vi "Get Array Values as JSON.vi"(8 "error in (no error)":errorcluster, 11 "JSON Array in":refnum<class "JSON Array.lvclass">) -> (0 "error out":errorcluster, 1 "single type?":bool, 2 "types":T1[](array[typedef]), 3 "values":refnum<class "JSON Null.lvclass">[](array[class]))   [LabVIEW 2016, in "LVJSON.lvlib" / "JSON Array.lvclass"]
doc: "Returns the element type of each element in a JSON Array. If all elements are of the same type, single type is true."
uses:
  JSON Array.lvclass
  JSON Types.ctl
  JSON Datatype/JSON Null.lvclass
  JSON Array.lvclass/JSON Array.ctl
  LVJSON.lvlib
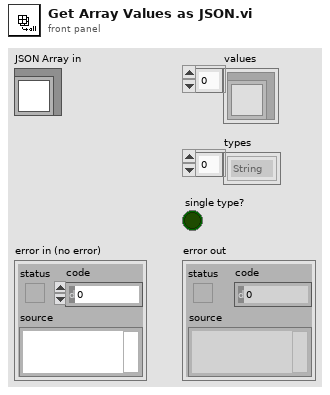
[diagram p1: front panel]
types:
  T1 = typedef "LVJSON.lvlib/JSON Types.ctl" = enum16{"String", "Numeric", "Boolean", "NULL", "Object", "Array"}
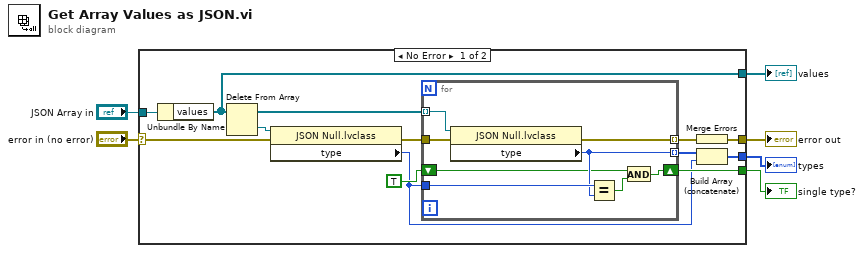
[diagram p0: block diagram]
diagram:
  n1 = case shown="No Error" "error in (no error)" {
    selector: "error in (no error)" -> [w11 w28]
    tunnel: [w8 w28] -> w5
    tunnel: "JSON Array in" -> [w19 _]
    tunnel: [w13 _] -> w3
    tunnel: [w15 _] -> w2
    tunnel: [w7 _] -> w1
    frame No Error {
      n2 = Unbundle By Name(w19) -> ("values"=w7:refnum<class "JSON Null.lvclass">[])
      n3 = Delete From Array(array=w7) -> (deleted portion=w18:refnum<class "JSON Null.lvclass">, array with subset deleted=w17:refnum<class "JSON Null.lvclass">[])  [unwired: 2 in]
      n4 = property class="JSON Null.lvclass"(reference=w18, error in=w11) -> (error out=w10:errorcluster, "type"=w12:T1)  [unwired: 1 out]
      n5 = for {
        tunnel: w17 -> [w27] mode=indexing
        tunnel: [w25] -> w14 mode=indexing
        tunnel: w12 -> [w26]
        shift-right: [w22] -> w15
        shift-left: TRUE -> [w23]
        tunnel: w10 -> [w21]
        tunnel: [w20] -> w9 mode=indexing
        n6 = property class="JSON Null.lvclass"(reference=w27, error in=w21) -> (error out=w20:errorcluster, "type"=w25:T1)  [unwired: 1 out]
        n7 = Equal?(x=w26, y=w25) -> (x = y?=w24:bool)
        n8 = And(x=w23, y=w24) -> (x .and. y?=w22:bool)
      }
      n9 = Merge Errors(w9) -> (w8:errorcluster)
      n10 = Build Array (concatenate)(w14, w12) -> (w13:T1[])
    }
    frame Error {
    }
  }
  "error out" <- w5
  "types" <- w3
  "single type?" <- w2
  "values" <- w1
